vi "M227.vi"(4 "Special Function In":string, 6 "Velocity":dbl, 7 "Abort":refnum<vi>, 8 "Axis":bool[](array[boolean]), 9 "Positions":dbl[](array[numeric]), 10 "Action":T1=enum."MVR", 11 "VISA In":refnum<visa-resource-name>) -> (0 "Special Function Out":string, 1 "Status":bool, 2 "Position Out":dbl[](array[numeric]), 3 "VISA Out":refnum<visa-resource-name>)   [LabVIEW 2014]
uses:
  Controls/StageStates.ctl
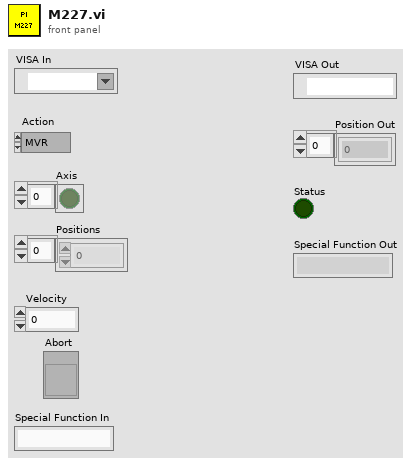
[diagram p1: front panel]
types:
  T1 = typedef "StageStates.ctl" = enum16{"POSITION", "MVR", "MOVE", "HALT", "ONTARGET", "ERROR", "EXIT", "HOME", "ZEROPOS", "NANOPOS", "QUIT", "ANALOG"}
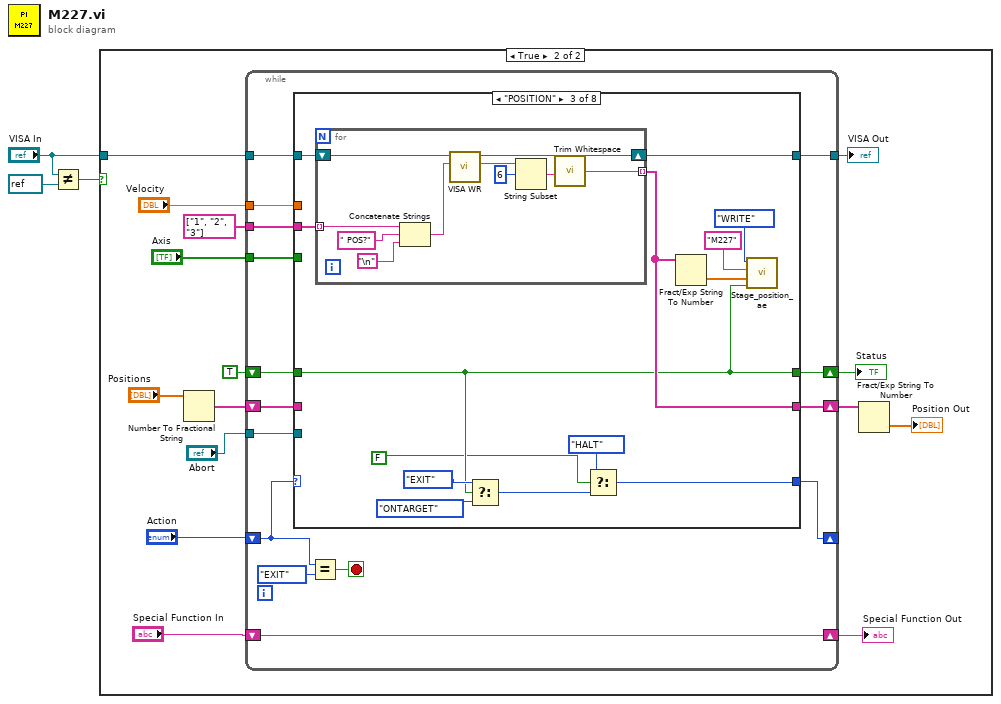
[diagram p0: block diagram]
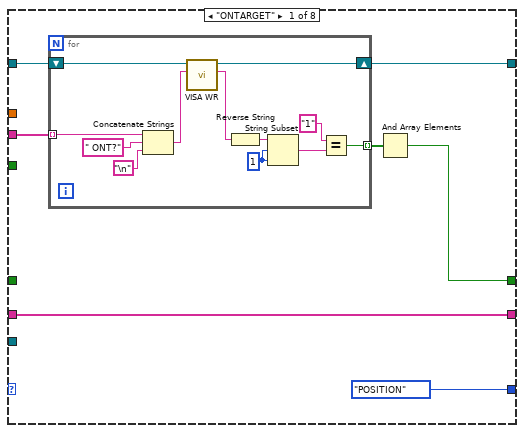
[diagram p3: hidden frame]
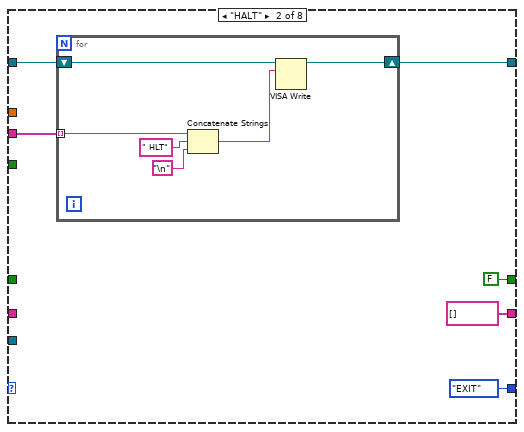
[diagram p4: hidden frame]
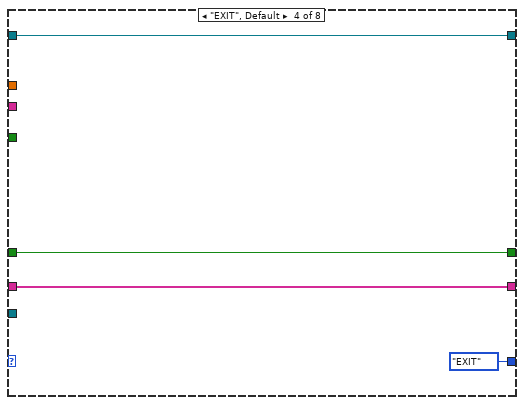
[diagram p5: hidden frame]
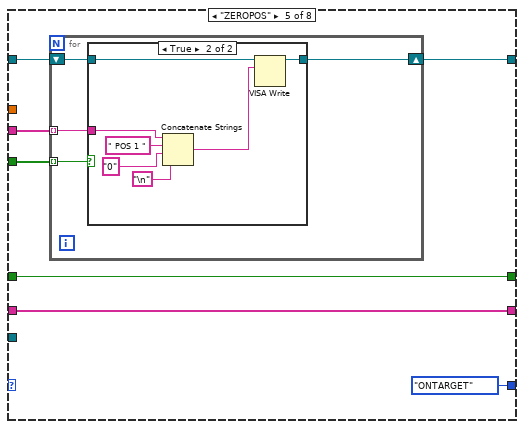
[diagram p6: hidden frame]
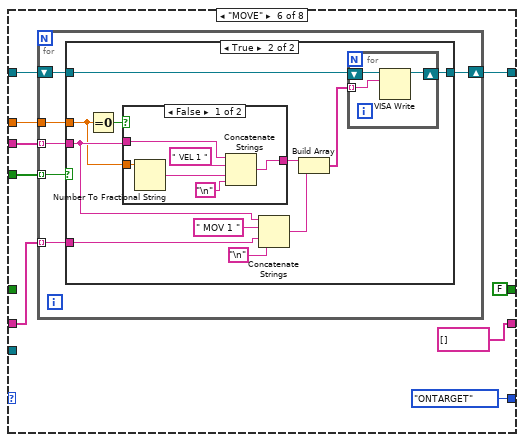
[diagram p8: hidden frame]
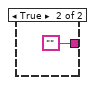
[diagram p10: hidden frame]
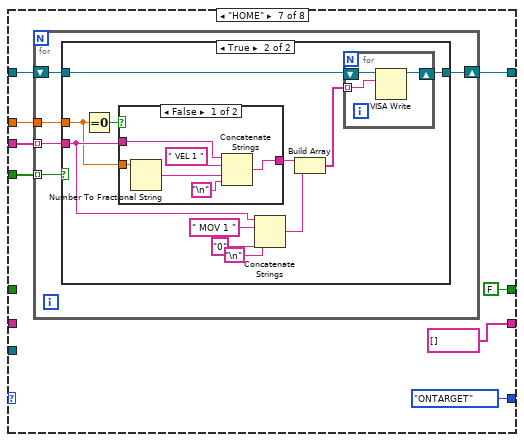
[diagram p11: hidden frame]
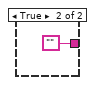
[diagram p13: hidden frame]
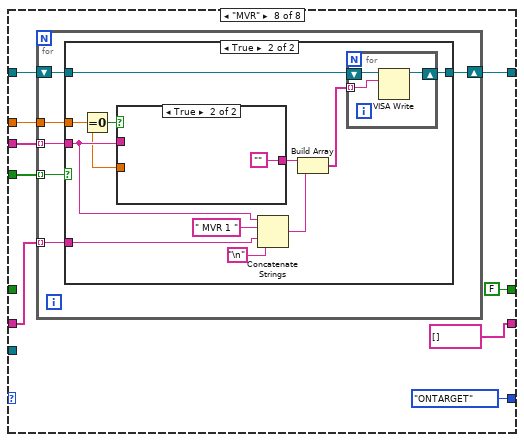
[diagram p14: hidden frame]
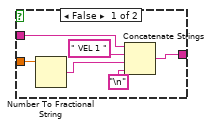
[diagram p16: hidden frame]
diagram:
  n1 = Not Equal?(x="VISA In", y=refnum<visa-resource-name> refnum ("VISA In")) -> (x != y?=w2:bool)
  n2 = case shown="True" w2 {
    tunnel: "VISA In" -> [_ w17]
    frame False {
    }
    frame True {
      n3 = Number To Fractional String(number="Positions") -> (F-format string=w11:string[])  [unwired: 3 in]
      n4 = while {
        tunnel: string[] ["1", "2", "3"] -> [w33]
        tunnel: w17 -> [w32]
        shift-right: [w22] -> _
        shift-left: "Action" -> [w27]
        shift-right: [w30] -> w9
        shift-left: w11 -> [w31]
        shift-right: [w28] -> w15
        shift-left: TRUE -> [w29]
        tunnel: "Axis" -> [w26]
        tunnel: "Velocity" -> [w25]
        shift-right: [w24] -> w7
        shift-left: "Special Function In" -> [w24]
        tunnel: [w21] -> w5
        tunnel: "Abort" -> [w19]
        stop <- w20 stop-if-true
        n5 = case shown="\"POSITION\"" w27 {
          tunnel: w33 -> [w39 w58 w77 _ w99 w120 w156 w192]
          tunnel: w32 -> [w40 w57 w78 w90 w98 w119 w155 w191]
          tunnel: w31 -> [w35 _ _ w92 w95 w118 _ w190]
          tunnel: [w35 string[] [] w72 w92 w95 string[] [] string[] [] string[] []] -> w30
          tunnel: w29 -> [_ _ w66 w91 w96 _ _ _]
          tunnel: [w37 FALSE w66 w91 w96 FALSE FALSE FALSE] -> w28
          tunnel: w26 -> [_ _ _ _ w97 w117 w154 w189]
          tunnel: w25 -> [_ _ _ _ _ w116 w153 w188]
          tunnel: [StageStates."POSITION" ("Action") StageStates."EXIT" ("Action") w69 StageStates."EXIT" ("Action") StageStates."ONTARGET" ("Action") StageStates."ONTARGET" ("Action") StageStates."ONTARGET" ("Action") StageStates."ONTARGET" ("Action")] -> w22
          tunnel: [w34 w53 w76 w90 w93 w114 w150 w184] -> w21
          tunnel: w19 -> [_ _ _ _ _ _ _ _]
          frame "ONTARGET" {
            n6 = for {
              tunnel: w39 -> [w51] mode=indexing
              tunnel: [w47] -> w38 mode=indexing
              shift-right: [w41] -> w34
              shift-left: w40 -> [w52]
              w43 = 1 ("length (rest)")
              n7 = Concatenate Strings(w51, " ONT?" ("string"), "\n") -> (w42:string)
              n8 = call "VISA WR.vi"("write buffer"=w42, "VISA Refnum in"=w52) -> ("read buffer"=w50:string, "VISA Refnum out"=w41:refnum<visa-resource-name>)  [unwired: 7 in, 1 out]
              n9 = Reverse String(1:w50) -> (0:w44:string)
              n10 = String Subset(string=w44, offset (0)=w43, length (rest)=w43) -> (substring=w49:string)
              n11 = Equal?(x="1", y=w49) -> (x = y?=w47:bool)
            }
            n12 = And Array Elements(Boolean array=w38) -> (logical AND=w37:bool)
          }
          frame "HALT" {
            n13 = for {
              tunnel: w58 -> [w63] mode=indexing
              shift-right: [w60] -> w53
              shift-left: w57 -> [w61]
              n14 = Concatenate Strings(w63, " HLT" ("string"), "\n") -> (w62:string)
              n15 = VISA Write(VISA resource name=w61, write buffer=w62) -> (VISA resource name out=w60:refnum<visa-resource-name>)  [unwired: 1 in, 2 out]
            }
          }
          frame "POSITION" {
            n16 = for {
              tunnel: w77 -> [w87] mode=indexing
              tunnel: [w85] -> w72 mode=indexing
              shift-right: [w79] -> w76
              shift-left: w78 -> [w88]
              n17 = Concatenate Strings(w87, " POS?" ("string"), "\n") -> (w80:string)
              n18 = call "VISA WR.vi"("write buffer"=w80, "VISA Refnum in"=w88) -> ("read buffer"=w86:string, "VISA Refnum out"=w79:refnum<visa-resource-name>)  [unwired: 7 in, 1 out]
              n19 = String Subset(string=w86, offset (0)=6) -> (substring=w81:string)  [unwired: 1 in]
              n20 = call <vilib>:"Trim Whitespace.vi"("string"=w81) -> ("trimmed string"=w85:string)  [unwired: 1 in]
            }
            n21 = Select(t=StageStates."EXIT" ("Action"), s=w66, f=StageStates."ONTARGET" ("Action")) -> (s? t:f=w67:T1)
            n22 = Select(t=StageStates."HALT" ("Action"), s=FALSE, f=w67) -> (s? t:f=w69:T1)
            n23 = Fract/Exp String To Number(string=w72) -> (number=w73:dbl[])  [unwired: 3 in, 1 out]
            n24 = call "Stage_position_ae.vi"("Status In"=w66, "Position In"=w73, "StageID"="M227", "Enum"=enum16{"WRITE", "READ"}."WRITE") -> ()  [unwired: 6 in, 2 out]
          }
          frame "EXIT", Default {
          }
          frame "ZEROPOS" {
            n25 = for {
              tunnel: w99 -> [w103] mode=indexing
              shift-right: [w101] -> w93
              shift-left: w98 -> [w102]
              tunnel: w97 -> [w100] mode=indexing
              n26 = case shown="True" w100 {
                tunnel: w103 -> [_ w108]
                tunnel: w102 -> [w104 w107]
                tunnel: [w104 w106] -> w101
                frame False {
                }
                frame True {
                  n27 = Concatenate Strings(w108, " POS 1 " ("string"), "0" ("f"), "\n") -> (w105:string)
                  n28 = VISA Write(VISA resource name=w107, write buffer=w105) -> (VISA resource name out=w106:refnum<visa-resource-name>)  [unwired: 1 in, 2 out]
                }
              }
            }
          }
          frame "MOVE" {
            n29 = for {
              tunnel: w120 -> [w126] mode=indexing
              tunnel: w118 -> [w125] mode=indexing
              shift-right: [w123] -> w114
              shift-left: w119 -> [w124]
              tunnel: w117 -> [w122] mode=indexing
              tunnel: w116 -> [w121]
              n30 = case shown="True" w122 {
                tunnel: w126 -> [_ w134]
                tunnel: w125 -> [_ w133]
                tunnel: w124 -> [w127 w137]
                tunnel: [w127 w136] -> w123
                tunnel: w121 -> [_ w128]
                frame False {
                }
                frame True {
                  n31 = Equal To 0?(x=w128) -> (x = 0?=w132:bool)
                  n32 = case shown="False" w132 {
                    tunnel: w134 -> [w145 _]
                    tunnel: [w144 ""] -> w131
                    tunnel: w128 -> [w142 _]
                    frame False {
                      n33 = Number To Fractional String(number=w142) -> (F-format string=w143:string)  [unwired: 3 in]
                      n34 = Concatenate Strings(w145, " VEL 1 ", w143, "\n") -> (w144:string)
                    }
                    frame True {
                    }
                  }
                  n35 = Concatenate Strings(w134, " MOV 1 ", w133, "\n") -> (w130:string)
                  n36 = Build Array(w131, w130) -> (w129:string[])
                  n37 = for {
                    shift-right: [w140] -> w136
                    shift-left: w137 -> [w141]
                    tunnel: w129 -> [w139] mode=indexing
                    n38 = VISA Write(VISA resource name=w141, write buffer=w139) -> (VISA resource name out=w140:refnum<visa-resource-name>)  [unwired: 1 in, 2 out]
                  }
                }
              }
            }
          }
          frame "HOME" {
            n39 = for {
              tunnel: w156 -> [w161] mode=indexing
              shift-right: [w159] -> w150
              shift-left: w155 -> [w160]
              tunnel: w154 -> [w158] mode=indexing
              tunnel: w153 -> [w157]
              n40 = case shown="True" w158 {
                tunnel: w161 -> [_ w169]
                tunnel: w160 -> [w162 w172]
                tunnel: [w162 w171] -> w159
                tunnel: w157 -> [_ w164]
                frame False {
                }
                frame True {
                  n41 = Equal To 0?(x=w164) -> (x = 0?=w168:bool)
                  n42 = case shown="False" w168 {
                    tunnel: w169 -> [w180 _]
                    tunnel: [w179 ""] -> w167
                    tunnel: w164 -> [w177 _]
                    frame False {
                      n43 = Number To Fractional String(number=w177) -> (F-format string=w178:string)  [unwired: 3 in]
                      n44 = Concatenate Strings(w180, " VEL 1 ", w178, "\n") -> (w179:string)
                    }
                    frame True {
                    }
                  }
                  n45 = Concatenate Strings(w169, " MOV 1 ", "0" ("string"), "\n") -> (w166:string)
                  n46 = Build Array(w167, w166) -> (w165:string[])
                  n47 = for {
                    shift-right: [w175] -> w171
                    shift-left: w172 -> [w176]
                    tunnel: w165 -> [w174] mode=indexing
                    n48 = VISA Write(VISA resource name=w176, write buffer=w174) -> (VISA resource name out=w175:refnum<visa-resource-name>)  [unwired: 1 in, 2 out]
                  }
                }
              }
            }
          }
          frame "MVR" {
            n49 = for {
              tunnel: w192 -> [w198] mode=indexing
              tunnel: w190 -> [w197] mode=indexing
              shift-right: [w195] -> w184
              shift-left: w191 -> [w196]
              tunnel: w189 -> [w194] mode=indexing
              tunnel: w188 -> [w193]
              n50 = case shown="True" w194 {
                tunnel: w198 -> [_ w206]
                tunnel: w197 -> [_ w205]
                tunnel: w196 -> [w199 w209]
                tunnel: [w199 w208] -> w195
                tunnel: w193 -> [_ w204]
                frame False {
                }
                frame True {
                  n51 = Equal To 0?(x=w204) -> (x = 0?=w203:bool)
                  n52 = case shown="True" w203 {
                    tunnel: w206 -> [w217 _]
                    tunnel: w204 -> [w215 _]
                    tunnel: [w216 ""] -> w202
                    frame False {
                      n53 = Number To Fractional String(number=w215) -> (F-format string=w214:string)  [unwired: 3 in]
                      n54 = Concatenate Strings(w217, " VEL 1 ", w214, "\n") -> (w216:string)
                    }
                    frame True {
                    }
                  }
                  n55 = Concatenate Strings(w206, " MVR 1 ", w205, "\n") -> (w201:string)
                  n56 = Build Array(w202, w201) -> (w200:string[])
                  n57 = for {
                    shift-right: [w212] -> w208
                    shift-left: w209 -> [w213]
                    tunnel: w200 -> [w211] mode=indexing
                    n58 = VISA Write(VISA resource name=w213, write buffer=w211) -> (VISA resource name out=w212:refnum<visa-resource-name>)  [unwired: 1 in, 2 out]
                  }
                }
              }
            }
          }
        }
        n59 = Equal?(x=w27, y=StageStates."EXIT") -> (x = y?=w20:bool)
      }
      "Status" <- w15
      "Special Function Out" <- w7
      "VISA Out" <- w5
      n60 = Fract/Exp String To Number(string=w9) -> (number=→"Position Out":dbl[])  [unwired: 3 in, 1 out]
    }
  }
